vi "read TBM configuration.vi"(8 "error in":errorcluster, 11 "TDMS datalogger editor node in":refnum<class "TDMS datalogger editor node.lvclass">) -> (0 "error out":errorcluster, 2 "configuration":refnum<class "TBM configuration.lvclass">, 3 "TDMS datalogger editor node out":refnum<class "TDMS datalogger editor node.lvclass">)   [LabVIEW 2013, in "TDMS datalogger editor node.lvclass"]
uses:
  TDMS datalogger editor node.lvclass
  <vilib>/NI/Tag Bus Module Framework/root configuration/TBM configuration.lvclass
  TDMS datalogger editor node.lvclass/TDMS datalogger editor node.ctl
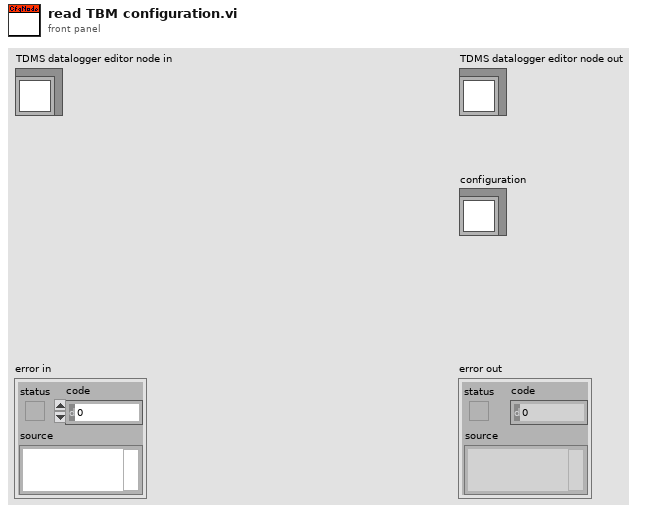
[diagram p1: front panel]
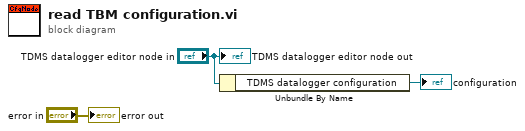
[diagram p0: block diagram]
diagram:
  n1 = Unbundle By Name("TDMS datalogger editor node in") -> ("TDMS datalogger configuration"=→"configuration":refnum<class "TDMS datalogger configuration.lvclass">)
  "error out" <- "error in"
  "TDMS datalogger editor node out" <- "TDMS datalogger editor node in"
